vi "Alicat Simple Terminal Interface.vi"() -> ()   [LabVIEW 2020]
doc: "Example VI for communicating with an Alicat through serial commands, similar to a serial terminal application such as HyperTerminal or PuTTY."
panel:
  in  "End Program":bool
  in  "COM Port Settings":T1={"Unit ID"="A", "Baud Rate"=enum."19200", "VISA Sesssion In"="COM1"}
  in  "OK Button":bool
  out "Response from Alicat":string
  in  "Command to Send":string
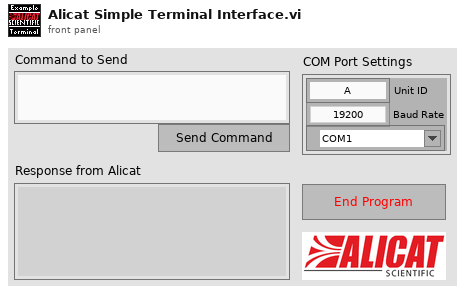
[diagram p1: front panel]
types:
  T1 = cluster{"Unit ID":string, "Baud Rate":enum8{"2400", "9600", "19200", "38400", "57600", "115200", "Unknown"}, "VISA Sesssion In":refnum<visa-resource-name>}
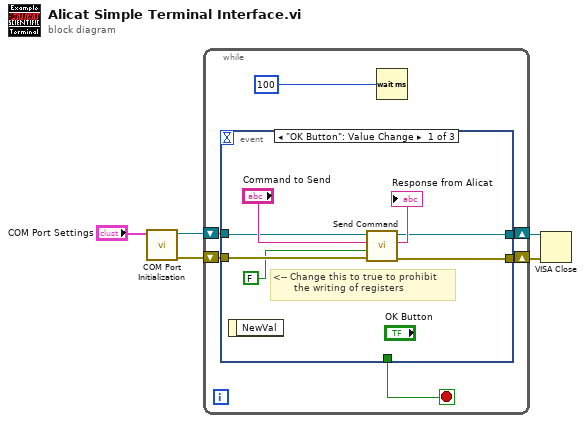
[diagram p0: block diagram]
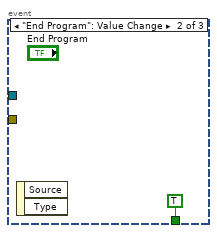
[diagram p2: hidden frame]
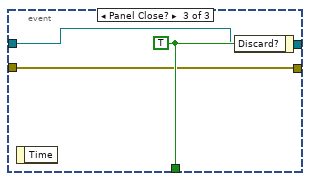
[diagram p3: hidden frame]
diagram:
  n1 = call "COM Port Initialization.vi"("Communication Settings"="COM Port Settings") -> ("error out"=w4:errorcluster, "VISA Session Out"=w5:refnum<visa-resource-name>)  [unwired: 9 in]
  n2 = while {
    shift-right: [w9] -> w3
    shift-left: w5 -> [w11]
    shift-right: [w8] -> w2
    shift-left: w4 -> [w10]
    stop <- w7 stop-if-true
    n3 = event shown="[0] \"OK Button\": Value Change" {
      selector: _ -> [_ _ _]
      dyn-events: _ -> [_ _ _]
      timeout: _ -> [_ _ _]
      tunnel: w11 -> [w14 _ w20]
      tunnel: w10 -> [w18 _ w21]
      tunnel: [w13 _ w20] -> w9
      tunnel: [w17 _ w21] -> w8
      tunnel: [_ TRUE ("Discard?") w22] -> w7
      event "OK Button": Value Change {
        # "<-- Change this to true to prohibit\n       the writing of registers"
        n4 = event-data() -> ()  [unwired: 1 in, 1 out]
        n5 = call "Send Command.vi"("error in"=w18, "Disable register writing (T)"=FALSE ("Disable register writing"), "Command"="Command to Send", "VISA Session In"=w14) -> ("error out"=w17:errorcluster, "Response"=→"Response from Alicat":string, "VISA Session Out"=w13:refnum<visa-resource-name>)  [unwired: 5 in]
      }
      event "End Program": Value Change {
        n6 = event-data() -> ()  [unwired: 1 in, 2 out]
      }
      event Panel Close? {
        w22 = TRUE ("Discard?")
        n7 = event-data() -> ()  [unwired: 1 in, 1 out]
        n8 = event-data("Discard?"=w22) -> ()  [unwired: 1 in, 1 out]
      }
    }
    n9 = Wait (ms)(milliseconds to wait=u32 100) -> ()  [unwired: 1 out]
  }
  n10 = VISA Close(VISA resource name=w3, error in (no error)=w2) -> ()  [unwired: 1 out]
